vi "digitally_ros_without_joystick_single_target.vi"() -> ()   [LabVIEW 2019]
uses:
  <vilib>/addons/eal4LabVIEW/ApiLib/Connection control/ealApiConnect_string.vi
  <vilib>/addons/eal4LabVIEW/eal4LabVIEW.lvlib
panel:
  out "Is the PID finished?":bool
  out "Iteration counter loop 1":i32
  out "Deviation 3":dbl
  out "Deviation 2":dbl
  out "Deviation 1":dbl
  out "Sensor values":dbl[](array[numeric])
  out "List length":i32
  in  "Loop 3":bool
  in  "Loop 2":bool
  out "Iteration counter loop 3":i32
  out "Initialization error":errorcluster
  out "In Range? (1)":bool
  out "In Range? (2)":bool
  out "In Range? (3)":bool
  in  "condition 6":i32(ring) items=["AXIS_CONDITION_ACTIVE"=0, "AXIS_CONDITION_PARKING"=1, "AXIS_CONDITION_DEACTIVATED"=2, "AXIS_CONDITION_ACTIVE_DECOUPLED"=4, "AXIS_CONDITION_PARKING_DECOUPLED"=5, "AXIS_CONDITION_DEACTIVATED_DECOUPLED"=6, "AXIS_CONDITION_ACTIVE_PARAMETERIZATION"=8, "AXIS_CONDITION_PARKING_PARAMETERIZATION"=9, "AXIS_CONDITION_DEACTIVATED_PARAMETERIZATION"=10, "AXIS_CONDITION_ACTIVE_DECOUPLED_PARAMETERIZATION"=12, "AXIS_CONDITION_PARKING_DECOUPLED_PARAMETERIZATION"=13, "AXIS_CONDITION_DEACTIVATED_DECOUPLED_PARAMETERIZATION"=14]
  in  "slave index 6":i32
  in  "condition 5":i32(ring) items=["AXIS_CONDITION_ACTIVE"=0, "AXIS_CONDITION_PARKING"=1, "AXIS_CONDITION_DEACTIVATED"=2, "AXIS_CONDITION_ACTIVE_DECOUPLED"=4, "AXIS_CONDITION_PARKING_DECOUPLED"=5, "AXIS_CONDITION_DEACTIVATED_DECOUPLED"=6, "AXIS_CONDITION_ACTIVE_PARAMETERIZATION"=8, "AXIS_CONDITION_PARKING_PARAMETERIZATION"=9, "AXIS_CONDITION_DEACTIVATED_PARAMETERIZATION"=10, "AXIS_CONDITION_ACTIVE_DECOUPLED_PARAMETERIZATION"=12, "AXIS_CONDITION_PARKING_DECOUPLED_PARAMETERIZATION"=13, "AXIS_CONDITION_DEACTIVATED_DECOUPLED_PARAMETERIZATION"=14]
  in  "slave index 5":i32
  in  "condition 4":i32(ring) items=["AXIS_CONDITION_ACTIVE"=0, "AXIS_CONDITION_PARKING"=1, "AXIS_CONDITION_DEACTIVATED"=2, "AXIS_CONDITION_ACTIVE_DECOUPLED"=4, "AXIS_CONDITION_PARKING_DECOUPLED"=5, "AXIS_CONDITION_DEACTIVATED_DECOUPLED"=6, "AXIS_CONDITION_ACTIVE_PARAMETERIZATION"=8, "AXIS_CONDITION_PARKING_PARAMETERIZATION"=9, "AXIS_CONDITION_DEACTIVATED_PARAMETERIZATION"=10, "AXIS_CONDITION_ACTIVE_DECOUPLED_PARAMETERIZATION"=12, "AXIS_CONDITION_PARKING_DECOUPLED_PARAMETERIZATION"=13, "AXIS_CONDITION_DEACTIVATED_DECOUPLED_PARAMETERIZATION"=14]
  in  "slave index 4":i32
  out "RPM Boom":dbl
  out "RPM Arm":dbl
  out "RPM Bucket":dbl
  in  "Loop 1":bool
  out "Return value":dbl[](array[numeric])
  out "Iteration counter loop 2":i32
  # "PID Control"
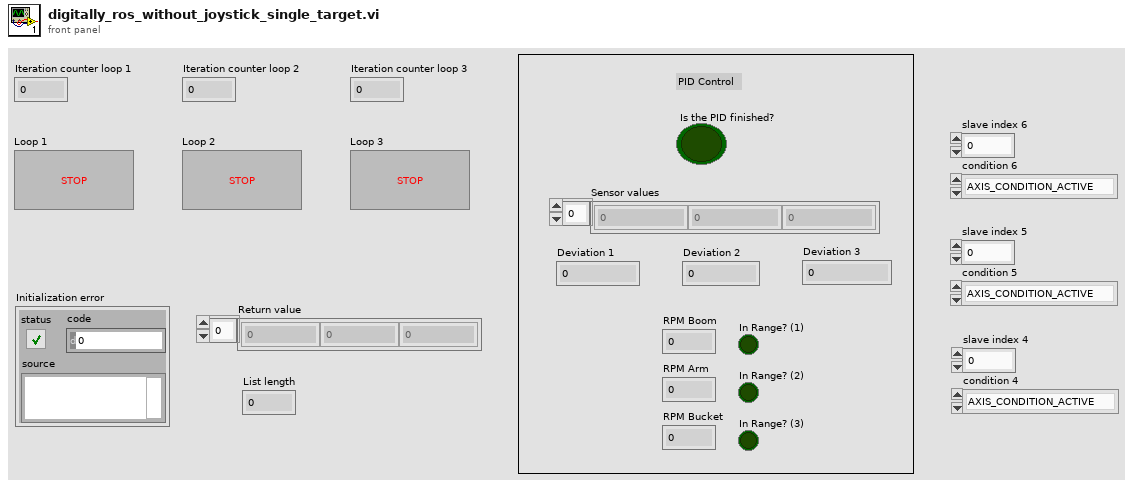
[diagram p1: front panel]
types:
  T1 = cluster{"Velocity":dbl, "Acceleration":dbl, "Deceleration":dbl, "Jerk":dbl}
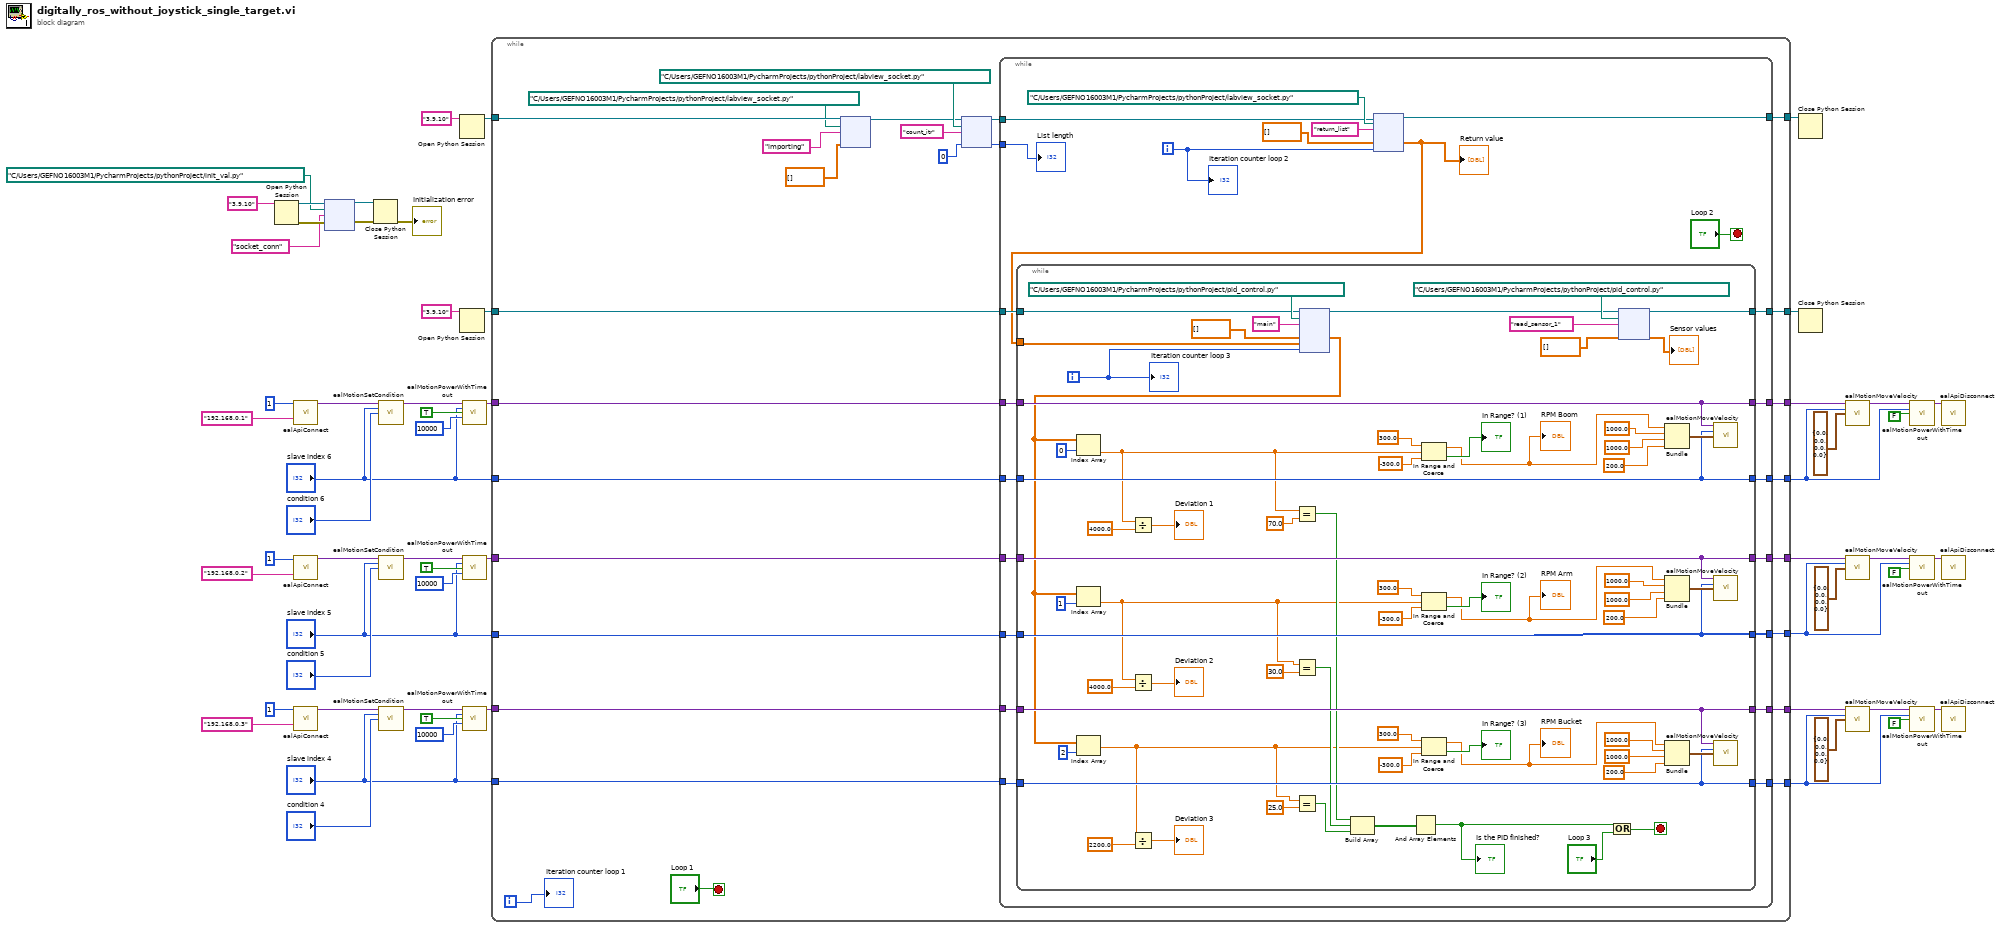
[diagram p0: block diagram]
diagram:
  n1 = Open Python Session(python version="3.9.10" ("Python version")) -> (session out=w9:refnum<k35>, error out=w7:errorcluster)  [unwired: 2 in]
  n2 = call-poly <vilib>:"ealApiConnect.vi"("maximum no of axes"=1, "ip address"="192.168.0.1") -> ("connection out"=w31:variant)  [unwired: 12 in, 1 out]
  n3 = call-poly <vilib>:"ealApiConnect.vi"("maximum no of axes"=1, "ip address"="192.168.0.2") -> ("connection out"=w38:variant)  [unwired: 12 in, 1 out]
  n4 = call-poly <vilib>:"ealApiConnect.vi"("maximum no of axes"=1, "ip address"="192.168.0.3") -> ("connection out"=w45:variant)  [unwired: 12 in, 1 out]
  n5 = node(w9, path "C:/Users/GEFNO16003M1/PycharmProjects/pythonProject/init_val.py" ("module path"), "socket_conn" ("function name"), w7) -> (w8:refnum<k35>, w6:errorcluster)  [unwired: 2 in, 2 out]
  n6 = Close Python Session(session in=w8, error in=w6) -> (11:→"Initialization error":errorcluster)
  n7 = call <vilib>:"ealMotionSetCondition.vi"("connection in"=w31, "slave index"="slave index 6", "condition"="condition 6") -> ("connection out"=w30:variant)  [unwired: 11 in, 1 out]
  n8 = call <vilib>:"ealMotionSetCondition.vi"("connection in"=w38, "slave index"="slave index 5", "condition"="condition 5") -> ("connection out"=w37:variant)  [unwired: 11 in, 1 out]
  n9 = call <vilib>:"ealMotionSetCondition.vi"("connection in"=w45, "slave index"="slave index 4", "condition"="condition 4") -> ("connection out"=w44:variant)  [unwired: 11 in, 1 out]
  n10 = Open Python Session(python version="3.9.10" ("Python version")) -> (session out=w16:refnum<k35>)  [unwired: 2 in, 1 out]
  n11 = Open Python Session(python version="3.9.10" ("Python version")) -> (session out=w13:refnum<k35>)  [unwired: 2 in, 1 out]
  n12 = call <vilib>:"ealMotionPowerWithTimeout.vi"("connection in"=w30, "slave index"="slave index 6", "value"=TRUE, "timeout"=10000) -> ("connection out"=w26:variant)  [unwired: 10 in, 1 out]
  n13 = call <vilib>:"ealMotionPowerWithTimeout.vi"("connection in"=w37, "slave index"="slave index 5", "value"=TRUE, "timeout"=10000) -> ("connection out"=w25:variant)  [unwired: 10 in, 1 out]
  n14 = call <vilib>:"ealMotionPowerWithTimeout.vi"("connection in"=w44, "slave index"="slave index 4", "value"=TRUE, "timeout"=10000) -> ("connection out"=w24:variant)  [unwired: 10 in, 1 out]
  n15 = while {
    tunnel: w26 -> [w85]
    tunnel: w25 -> [w84]
    tunnel: w24 -> [w83]
    tunnel: [w70] -> w23
    tunnel: [w82] -> w1
    tunnel: "slave index 6" -> [w81]
    tunnel: "slave index 5" -> [w80]
    tunnel: [w79] -> w20
    tunnel: [w73] -> w19
    tunnel: "slave index 4" -> [w78]
    tunnel: w16 -> [w77]
    tunnel: [w76] -> w15
    tunnel: w13 -> [w75]
    tunnel: [w71] -> w12
    tunnel: [w74] -> w11
    tunnel: [w72] -> w10
    i -> [w60]
    stop <- "Loop 1" stop-if-true
    n16 = node(w77, path "C:/Users/GEFNO16003M1/PycharmProjects/pythonProject/labview_socket.py" ("module path"), "importing" ("function name"), dbl[] []) -> (w64:refnum<k35>)  [unwired: 2 in, 3 out]
    n17 = node(w64, path "C:/Users/GEFNO16003M1/PycharmProjects/pythonProject/labview_socket.py" ("module path"), "count_itr" ("function name"), 0) -> (w63:refnum<k35>, w61:i32)  [unwired: 1 in, 3 out]
    n18 = while {
      tunnel: [w105] -> w76
      tunnel: w63 -> [w107]
      tunnel: w61 -> [w88]
      tunnel: w85 -> [w104]
      tunnel: w84 -> [w93]
      tunnel: w83 -> [w103]
      tunnel: [w95] -> w70
      tunnel: [w96] -> w82
      tunnel: w81 -> [w94]
      tunnel: w80 -> [w92]
      tunnel: [w97] -> w79
      tunnel: w78 -> [w99]
      tunnel: w75 -> [w91]
      tunnel: [w101] -> w71
      tunnel: [w100] -> w74
      tunnel: [w98] -> w73
      tunnel: [w90] -> w72
      i -> [w102]
      stop <- "Loop 2" stop-if-true
      n19 = node(w107, path "C:/Users/GEFNO16003M1/PycharmProjects/pythonProject/labview_socket.py" ("module path"), "return_list" ("function name"), dbl[] [], w102) -> (w105:refnum<k35>, w87:dbl[])  [unwired: 2 in, 3 out]
      "Return value" <- w87
      n20 = while {
        tunnel: w87 -> [w128]
        tunnel: w104 -> [w145]
        tunnel: w103 -> [w147]
        tunnel: [w147] -> w101
        tunnel: [w146] -> w100
        tunnel: w99 -> [w146]
        tunnel: [w143] -> w98
        tunnel: [w142] -> w97
        tunnel: [w144] -> w96
        tunnel: [w145] -> w95
        tunnel: w94 -> [w144]
        tunnel: w93 -> [w143]
        tunnel: w92 -> [w142]
        tunnel: w91 -> [w141]
        tunnel: [w127] -> w90
        i -> [w115]
        stop <- w130 stop-if-true
        n21 = node(w141, path "C:/Users/GEFNO16003M1/PycharmProjects/pythonProject/pid_control.py" ("module path"), "main" ("function name"), dbl[] [], w128, w115) -> (w122:refnum<k35>, w140:dbl[])  [unwired: 3 in, 3 out]
        n22 = Index Array(array=w140, index=0) -> (element=w110:dbl)
        n23 = Index Array(array=w140, index=1) -> (element=w111:dbl)
        n24 = Index Array(array=w140, index=2) -> (element=w112:dbl)
        n25 = Divide(x=w110, y=4000.0) -> (x/y=→"Deviation 1":dbl)
        n26 = Divide(x=w111, y=4000.0) -> (x/y=→"Deviation 2":dbl)
        n27 = Divide(x=w112, y=2200.0) -> (x/y=→"Deviation 3":dbl)
        n28 = Equal?(x=w110, y=70.0) -> (x = y?=w136:bool)
        n29 = Equal?(x=w111, y=30.0) -> (x = y?=w135:bool)
        n30 = Equal?(x=w112, y=25.0) -> (x = y?=w134:bool)
        n31 = Build Array(w136, w135, w134) -> (w114:bool[])
        n32 = And Array Elements(Boolean array=w114) -> (logical AND=w113:bool)
        "Is the PID finished?" <- w113
        n33 = In Range and Coerce(upper limit=300.0, x=w110, lower limit=-300.0) -> (coerced(x)=w133:dbl, In Range?=→"In Range? (1)":bool)
        "RPM Boom" <- w133
        n34 = In Range and Coerce(upper limit=300.0, x=w111, lower limit=-300.0) -> (coerced(x)=w132:dbl, In Range?=→"In Range? (2)":bool)
        "RPM Arm" <- w132
        n35 = In Range and Coerce(upper limit=300.0, x=w112, lower limit=-300.0) -> (coerced(x)=w131:dbl, In Range?=→"In Range? (3)":bool)
        "RPM Bucket" <- w131
        n36 = Or(x=w113, y="Loop 3") -> (x .or. y?=w130:bool)
        n37 = node(w122, path "C:/Users/GEFNO16003M1/PycharmProjects/pythonProject/pid_control.py" ("module path"), "read_sensor_1" ("function name"), dbl[] []) -> (w127:refnum<k35>, →"Sensor values":dbl[])  [unwired: 1 in, 3 out]
        n38 = Bundle("upper limit"=w133, 1000.0, 1000.0, 200.0) -> (w157:cluster{"upper limit":dbl, dbl, dbl, dbl})  [unwired: 1 in]
        n39 = Bundle("upper limit"=w132, 1000.0, 1000.0, 200.0) -> (w162:cluster{"upper limit":dbl, dbl, dbl, dbl})  [unwired: 1 in]
        n40 = Bundle("upper limit"=w131, 1000.0, 1000.0, 200.0) -> (w167:cluster{"upper limit":dbl, dbl, dbl, dbl})  [unwired: 1 in]
        n41 = call <vilib>:"ealMotionMoveVelocity.vi"("connection in"=w145, "slave index"=w144, "parameters set"=w157) -> ()  [unwired: 11 in, 2 out]
        n42 = call <vilib>:"ealMotionMoveVelocity.vi"("connection in"=w143, "slave index"=w142, "parameters set"=w162) -> ()  [unwired: 11 in, 2 out]
        n43 = call <vilib>:"ealMotionMoveVelocity.vi"("connection in"=w147, "slave index"=w146, "parameters set"=w167) -> ()  [unwired: 11 in, 2 out]
        "Iteration counter loop 3" <- w115
      }
      "Iteration counter loop 2" <- w102
      "List length" <- w88
    }
    "Iteration counter loop 1" <- w60
  }
  n44 = Close Python Session(session in=w15) -> ()  [unwired: 1 in, 1 out]
  n45 = Close Python Session(session in=w10) -> ()  [unwired: 1 in, 1 out]
  n46 = call <vilib>:"ealMotionMoveVelocity.vi"("connection in"=w23, "slave index"=w1, "parameters set"=T1 {"Velocity"=0.0, "Acceleration"=0.0, "Deceleration"=0.0, "Jerk"=0.0}) -> ("connection out"=w50:variant)  [unwired: 11 in, 1 out]
  n47 = call <vilib>:"ealMotionMoveVelocity.vi"("connection in"=w19, "slave index"=w20, "parameters set"=T1 {"Velocity"=0.0, "Acceleration"=0.0, "Deceleration"=0.0, "Jerk"=0.0}) -> ("connection out"=w54:variant)  [unwired: 11 in, 1 out]
  n48 = call <vilib>:"ealMotionMoveVelocity.vi"("connection in"=w12, "slave index"=w11, "parameters set"=T1 {"Velocity"=0.0, "Acceleration"=0.0, "Deceleration"=0.0, "Jerk"=0.0}) -> ("connection out"=w58:variant)  [unwired: 11 in, 1 out]
  n49 = call <vilib>:"ealMotionPowerWithTimeout.vi"("connection in"=w50, "slave index"=w1, "value"=FALSE) -> ("connection out"=w51:variant)  [unwired: 11 in, 1 out]
  n50 = call <vilib>:"ealMotionPowerWithTimeout.vi"("connection in"=w54, "slave index"=w20, "value"=FALSE) -> ("connection out"=w55:variant)  [unwired: 11 in, 1 out]
  n51 = call <vilib>:"ealMotionPowerWithTimeout.vi"("connection in"=w58, "slave index"=w11, "value"=FALSE) -> ("connection out"=w59:variant)  [unwired: 11 in, 1 out]
  n52 = call <vilib>:"ealApiDisconnect.vi"("connection in"=w51) -> ()  [unwired: 14 in, 1 out]
  n53 = call <vilib>:"ealApiDisconnect.vi"("connection in"=w55) -> ()  [unwired: 14 in, 1 out]
  n54 = call <vilib>:"ealApiDisconnect.vi"("connection in"=w59) -> ()  [unwired: 14 in, 1 out]
